vi "GetDigitalInputStatus.vi"(0 "VISA resource name":refnum<visa-resource-name>, 11 "error in":errorcluster) -> (4 "VISA resource name out":refnum<visa-resource-name>, 6 "Digital Input Status string":string, 8 "Digital Input Status":i32, 10 "Digital Input Status binary":string, 15 "error out":errorcluster)   [LabVIEW 2023, in "Thermotron 8800.lvlib"]
doc: "DIGI\nCommand name: Send digital input (DI) status\nCommand type: System status\nDescription: This command returns a 24-bit integer value that indicates which digital inputs are active.\nBits 0 through 23:\n0 through 5 CM0 digital inputs 1 through 6\n6 through 11 CM1 digital inputs 1 through 6\n12 through 17 CM2 digital inputs 1 through 6\n18 through 23 CM3 digital inputs 1 through 6\nDI 6 DI 5 DI 4 DI 3 DI 2 DI 1 CM\nbit 5 bit 4 bit 3 bit 2 bit 1 bit 0 0\nbit 11 bit 10 bit 9 bit 8 bit 7 bit 6 1\nbit 17 bit 16 bit 15 bit 14 bit 13 bit 12 2\nbit 23 bit 22 bit 21 bit 20 bit 19 bit 18 3\nQuery example 1: DIGI?\n8800 response: 0 (No digital inputs are active.)\nQuery example 2: DIGI?\n8800 response: 58498 =\n000000 001110 010010 000010\n CM3 CM2 CM1 CM0\nDI 6 DI 5 DI 4 DI 3 DI 2 DI 1 CM\nbit 5: 0 bit 4: 0 bit 3: 0 bit 2: 0 bit 1: 1 bit 0: 0 0\n(CM0 digital input 2, CM1 digital inputs 2 and 5, and CM2 digital inputs 2, 3, and 4 are\nactive.)"
uses:
  Thermotron 8800.lvlib
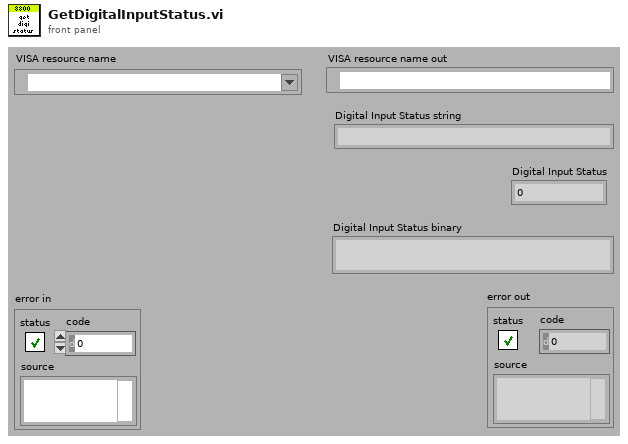
[diagram p1: front panel]
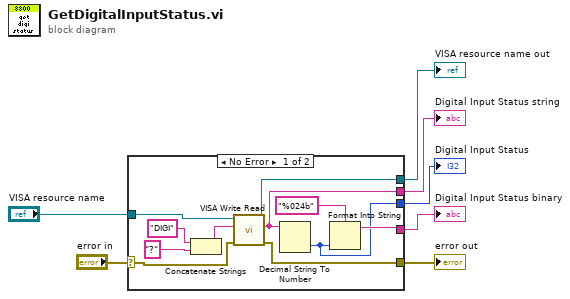
[diagram p0: block diagram]
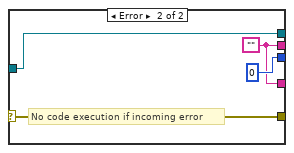
[diagram p2: hidden frame]
diagram:
  n1 = case shown="No Error" "error in" {
    selector: "error in" -> [w16 w22]
    tunnel: [w15 w22] -> w5
    tunnel: "VISA resource name" -> [w14 w20]
    tunnel: [w13 w20] -> w4
    tunnel: [w12 w19] -> w3
    tunnel: [w8 0] -> w2
    tunnel: [w9 w19] -> w1
    frame No Error {
      n2 = Concatenate Strings("DIGI" ("8800 Command"), "?" ("8800 Command")) -> (w18:string)
      n3 = call "VISA Write Read.vi"("error in (no error)"=w16, "8800 Command"=w18, "VISA Refnum in"=w14) -> ("error out"=w15:errorcluster, "read buffer"=w12:string, "VISA Refnum out"=w13:refnum<visa-resource-name>)  [unwired: 6 in]
      n4 = Decimal String To Number(string=w12) -> (number=w8:i32)  [unwired: 2 in, 1 out]
      n5 = Format Into String(format string="%024b", w8) -> (resulting string=w9:string)  [unwired: 2 in, 1 out]
    }
    frame Error {
      w19 = ""
      # "No code execution if incoming error"
    }
  }
  "VISA resource name out" <- w4
  "error out" <- w5
  "Digital Input Status string" <- w3
  "Digital Input Status" <- w2
  "Digital Input Status binary" <- w1
